vi "Brute Force Dark Current Primary Logic Body.vi"(0 "Barcodes in":string[](array[string]), 1 "stop":bool, 2 "Pins In":refnum<k21>[](array[refnum]), 5 "VISA Refnum in":refnum<visa-resource-name>, 6 "Number of Tubes":i32, 7 "Channel #":i32) -> (10 "Actual Voltage Level (V)":dbl format="%#_13g", 11 "Individual Tube Current (Nano Amps)":dbl[](array[numeric]), 12 "Actual Current Limit (nA)":dbl format="%#_13g", 13 "Mesurnment  Iteration":i32, 14 "Power Supply Trip":bool, 16 "Pins Out":refnum<k21>[](array[refnum]), 19 "Failed Tubes":string[](array[string]))   [LabVIEW 2020]
uses:
  <instrlib>/CAEN PSM/CAEN PSM.lvlib
panel:
  out "error out":errorcluster
  in  "First Tube #":i32
  out "BoardHandle out":T1
  # "Pin in"
  # "Pin out"
  # "No pin"
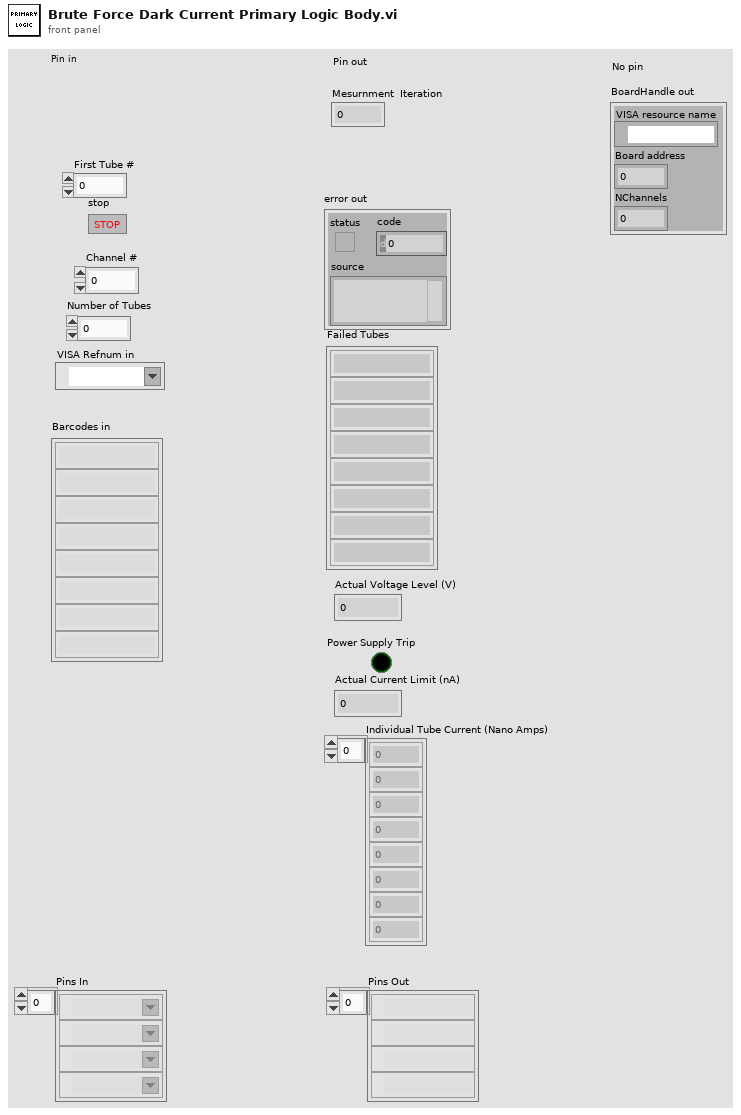
[diagram p1: front panel]
types:
  T1 = cluster{"VISA resource name":refnum<visa-resource-name>, "Board address":u8, "NChannels":u8}
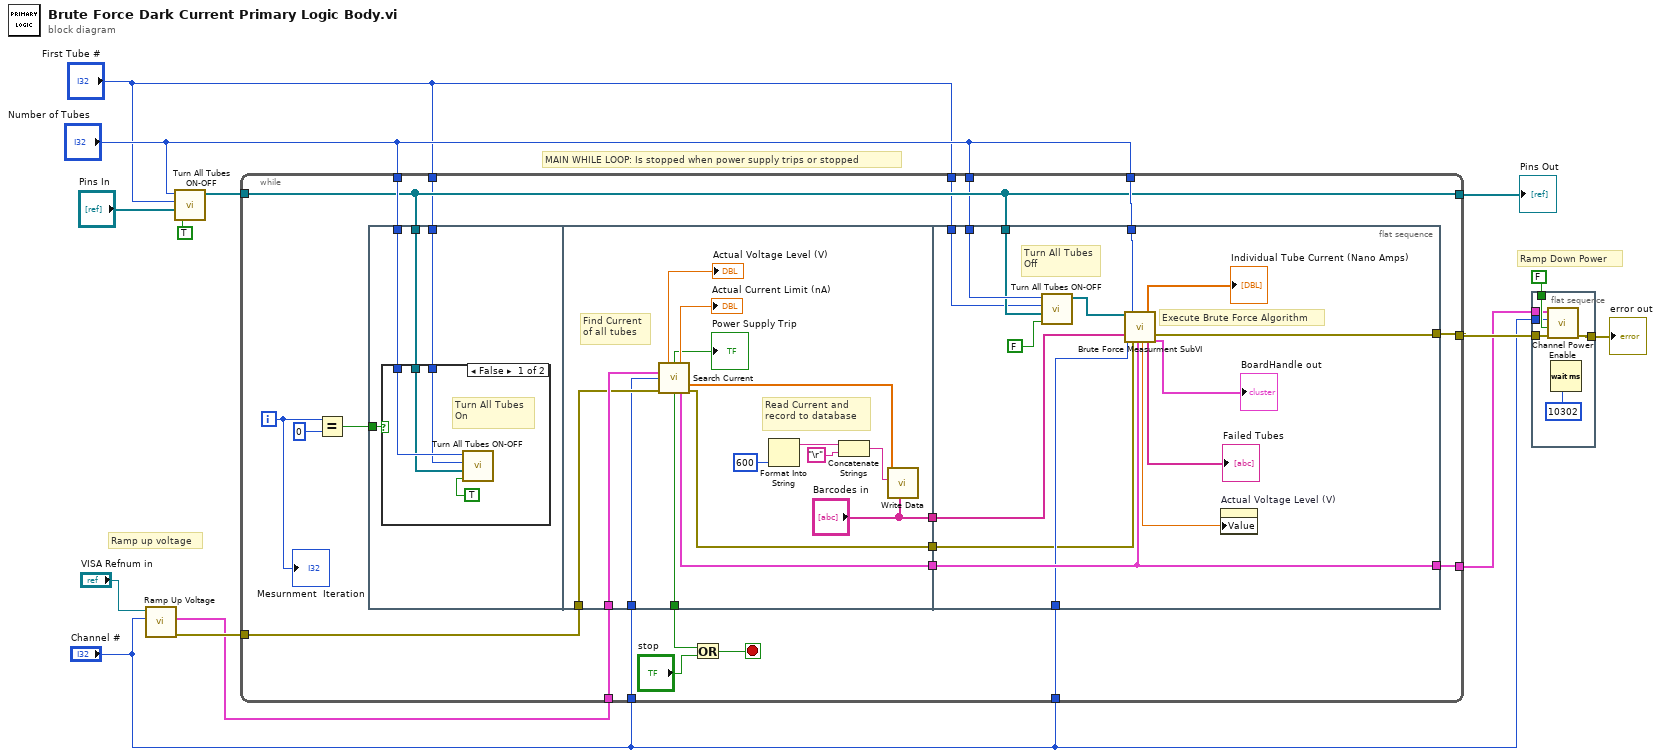
[diagram p0: block diagram]
diagram:
  # "Ramp Down Power"
  # "MAIN WHILE LOOP: Is stopped when power supply trips or stopped"
  # "Ramp up voltage"
  n1 = call "Ramp Up Voltage.vi"("Channel # in"="Channel #", "VISA Refnum in"="VISA Refnum in") -> ("error out"=w11:errorcluster, "BoardHandle out"=w10:T1)  [unwired: 8 in]
  n2 = call "Turn All Tubes ON-OFF.vi"("Activate: 1\nDeactivate: 0"=TRUE ("Activate: 1\nDeactivate: 0"), "Pins In"="Pins In", "First Tube #"="First Tube #", "Last Tube #"="Number of Tubes") -> ("Pins Out"=w4:refnum<k21>[])  [unwired: 7 in]
  n3 = while {
    tunnel: "Number of Tubes" -> [w35]
    tunnel: "Number of Tubes" -> [w20]
    tunnel: "Channel #" -> [w34]
    tunnel: w10 -> [w33]
    tunnel: "Number of Tubes" -> [w32]
    tunnel: w11 -> [w28]
    tunnel: [w24] -> w12
    tunnel: [w23] -> w14
    tunnel: w4 -> [w21]
    tunnel: "Channel #" -> [w22]
    tunnel: [w21] -> w7
    tunnel: "First Tube #" -> [w16]
    tunnel: "First Tube #" -> [w15]
    i -> [w19]
    stop <- w26 stop-if-true
    n4 = Equal?(x=w19, y=0) -> (x = y?=w17:bool)
    n5 = flat-sequence {
      tunnel: w32 -> [w39]
      tunnel: w21 -> [w38]
      tunnel: w17 -> [w37]
      tunnel: w16 -> [w36]
      tunnel: w34 -> [w46]
      tunnel: w33 -> [w49]
      tunnel: [w53] -> w31
      tunnel: [w51] -> w30
      tunnel: ["Barcodes in"] -> w29
      tunnel: w28 -> [w48]
      tunnel: [w45] -> w27
      tunnel: w35 -> [w71]
      tunnel: w29 -> [w72]
      tunnel: w30 -> [w70]
      tunnel: w31 -> [w61]
      tunnel: w20 -> [w65]
      tunnel: [w70] -> w24
      tunnel: [w60] -> w23
      tunnel: w22 -> [w63]
      tunnel: w21 -> [w62]
      tunnel: w15 -> [w58]
      frame #0 {
        n6 = case shown="False" w37 {
          tunnel: w39 -> [w43 _]
          tunnel: w38 -> [w41 _]
          tunnel: w36 -> [w40 _]
          frame False {
            # "Turn All Tubes \nOn"
            n7 = call "Turn All Tubes ON-OFF.vi"("Activate: 1\nDeactivate: 0"=TRUE, "Pins In"=w41, "First Tube #"=w40, "Last Tube #"=w43) -> ()  [unwired: 7 in, 1 out]
          }
          frame True {
          }
        }
      }
      frame #1 {
        # "Find Current\nof all tubes"
        # "Read Current and  record to database"
        n8 = call "Search Current.vi"("BoardHandle in"=w49, "Channel # in"=w46, "error in (no error)"=w48) -> ("Actual Voltage Level (V)"=→"Actual Voltage Level (V)":dbl, "Power Supply Trip"=w45:bool, "Actual Current Limit (nA)"=→"Actual Current Limit (nA)":dbl, "Array"=w52:dbl[], "BoardHandle out 2"=w51:T1, "error out"=w53:errorcluster)  [unwired: 7 in]
        "Power Supply Trip" <- w45
        n9 = Format Into String(600 ("input 1")) -> (resulting string=w56:string)  [unwired: 3 in, 1 out]
        n10 = Concatenate Strings(w56, "\r") -> (w57:string)
        n11 = call "Write Data.vi"("Barcodes"="Barcodes in", "Array"=w52, "String"=w57) -> ()  [unwired: 9 in]
      }
      frame #2 {
        # "Execute Brute Force Algorithm"
        # "Turn All Tubes\nOff"
        n12 = call "Turn All Tubes ON-OFF.vi"("Activate: 1\nDeactivate: 0"=FALSE ("Activate: 1\nDeactivate: 0"), "Pins In"=w62, "First Tube #"=w58, "Last Tube #"=w65) -> ("Pins Out"=w59:refnum<k21>[])  [unwired: 7 in]
        n13 = call "Brute Force Measurment SubVI.vi"("Pins In"=w59, "Barcodes in"=w72, "Channel # in"=w63, "Last Tube #"=w71, "error in (no error)"=w61, "BoardHandle in"=w70) -> ("Actual Voltage Level (V) 2"=w69:dbl, "Individual Tube Current (Nano Amps)"=→"Individual Tube Current (Nano Amps)":dbl[], "Failed Tubes"=→"Failed Tubes":string[], "error out"=w60:errorcluster, "BoardHandle out"=→"BoardHandle out":T1)  [unwired: 8 in, 1 out]
        n14 = property on="Actual Voltage Level (V)" class="DigNum (strict)"("Value"=w69) -> ()  [unwired: 2 in, 2 out]
      }
    }
    n15 = Or(x=w27, y="stop") -> (x .or. y?=w26:bool)
    "Mesurnment  Iteration" <- w19
  }
  "Pins Out" <- w7
  n16 = flat-sequence {
    tunnel: w14 -> [w78]
    tunnel: FALSE ("Enable (OFF)") -> [w77]
    tunnel: w12 -> [w76]
    tunnel: "Channel #" -> [w75]
    tunnel: [w74] -> w6
    frame #0 {
      n17 = call <instrlib>:"Channel Power Enable.vi"("error in (no error)"=w78, "Enable (OFF)"=w77, "Channel (0)"=w75, "BoardHandle"=w76) -> ("error out"=w74:errorcluster)  [unwired: 6 in, 1 out]
      n18 = Wait (ms)(milliseconds to wait=u32 10302) -> ()  [unwired: 1 out]
    }
  }
  "error out" <- w6
